vi "FGV_Logs.vi"(7 "Logs Action (GetList)":T2=enum."GetList", 8 "error in (no error)":errorcluster, 10 "Record Number":i32, 11 "Log":T1) -> (0 "error out":errorcluster, 3 "Logs":string)   [LabVIEW 2020]
uses:
  #typedef_FGV_LogsAction.ctl
  #typedef_Log.ctl
  #typedef_LogsData.ctl
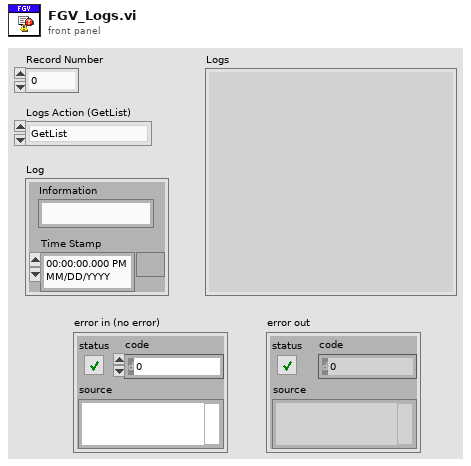
[diagram p1: front panel]
types:
  T1 = typedef "#typedef_Log.ctl" = cluster{"Information":string, "Time Stamp":timestamp}
  T2 = typedef "#typedef_FGV_LogsAction.ctl" = enum16{"ClearList", "AddRecord", "GetList"}
  T3 = typedef "#typedef_LogsData.ctl" = T1[]
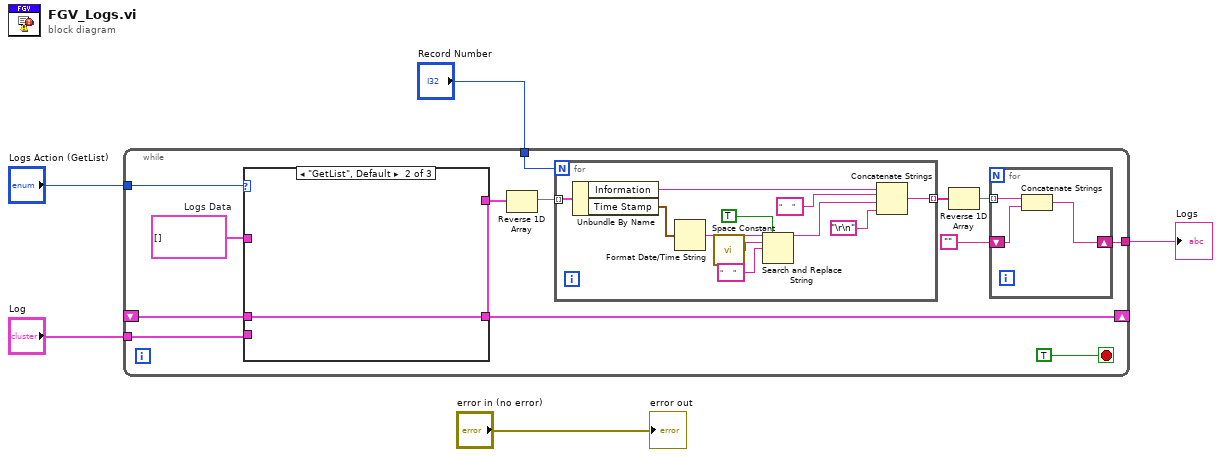
[diagram p0: block diagram]
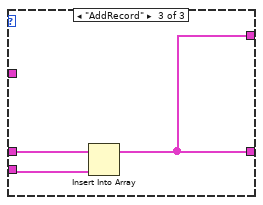
[diagram p3: hidden frame]
diagram:
  n1 = while {
    tunnel: "Logs Action (GetList)" -> [w17]
    tunnel: "Log" -> [w13]
    shift-right: [w15] -> _
    shift-left: _ -> [w14]
    tunnel: "Record Number" -> [w12]
    tunnel: [w8] -> w5
    stop <- TRUE stop-if-true
    w16 = T3 []  # Logs Data
    n2 = case shown="\"GetList\", Default" w17 {
      tunnel: w16 -> [w33 _ _]
      tunnel: [w33 w34 w35] -> w15
      tunnel: [w33 w34 w35] -> w11
      tunnel: w14 -> [_ w34 w37]
      tunnel: w13 -> [_ _ w36]
      frame "ClearList" {
      }
      frame "GetList", Default {
      }
      frame "AddRecord" {
        n3 = Insert Into Array(array=w37, new element=w36) -> (w35:T3)  [unwired: 1 in]
      }
    }
    n4 = Reverse 1D Array(array=w11) -> (reversed array=w10:T3)
    n5 = for {
      N: w12 -> [_]
      tunnel: w10 -> [w32] mode=indexing
      tunnel: [w23] -> w9 mode=indexing
      n6 = Unbundle By Name(w32) -> ("Information"=w30:string, "Time Stamp"=w31:timestamp)
      n7 = Format Date/Time String(seconds (now)=w31) -> (date/time string=w25:string)  [unwired: 2 in]
      n8 = call <vilib>:"Space Constant.vi"() -> ("String"=w28:string)
      n9 = Search and Replace String(replace all?=TRUE ("replace all? (F)"), input string=w25, search string=w28, replace string="     " ("replace string (\"\")")) -> (result string=w24:string)  [unwired: 4 in, 3 out]
      n10 = Concatenate Strings(w30, "     " ("replace string (\"\")"), w24, "\r\n") -> (w23:string)
    }
    n11 = Reverse 1D Array(array=w9) -> (reversed array=w6:string[])
    n12 = for {
      tunnel: w6 -> [w21] mode=indexing
      shift-right: [w20] -> w8
      shift-left: "" -> [w19]
      n13 = Concatenate Strings(w21, w19) -> (w20:string)
    }
  }
  "Logs" <- w5
  "error out" <- "error in (no error)"
